vi "Fitting on a Sphere.vi"(3 "Z":dbl[](array[numeric]) format="%.2f", 4 "Y":dbl[](array[numeric]) format="%.2f", 5 "X":dbl[](array[numeric]) format="%.2f") -> (0 "error":i32, 1 "r":dbl format="%.2f", 2 "x0, y0, z0":dbl[](array[numeric]) format="%.2f")   [LabVIEW 2017, in "NI_Gmath.lvlib"]
doc: "Determines the best spherical fit on a cloud of points in 3D."
uses:
  <vilib>/gmath/NI_Gmath.lvlib
  <vilib>/Analysis/baseanly.llb/Mean (DBL).vi
  <vilib>/Analysis/7linalg.llb/Solve Linear Equations (single right hand).vi
  <vilib>/Analysis/baseanly.llb/Solve Linear Equations By Cholesky.vi
  <vilib>/Analysis/baseanly.llb/Real Matrix to Compact Array.vi
  <vilib>/Analysis/baseanly.llb/Real Compact Tri-Matrix Linear Eqs.vi
  <vilib>/Analysis/7linalg.llb/Solve Linear Eqs (General).vi
  <vilib>/Analysis/7linalg.llb/Solve Linear Eqs (Gen, single right hand).vi
  <vilib>/Analysis/NI_AALPro.lvlib
  <vilib>/Analysis/NI_AALBase.lvlib
panel:
  # "Example:\n\n X: data points\n Y: data points \n Z: data points"
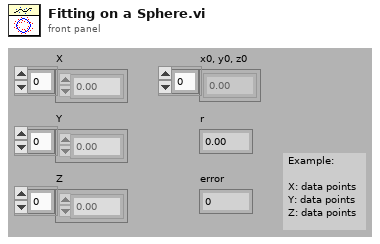
[diagram p1: front panel]
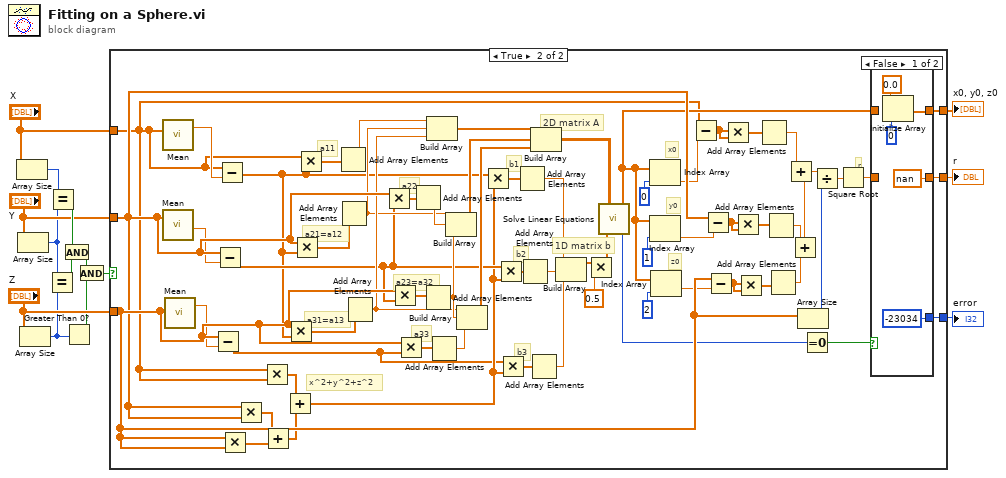
[diagram p0: block diagram]
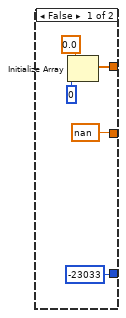
[diagram p2: hidden frame]
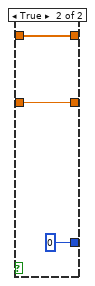
[diagram p3: hidden frame]
diagram:
  n1 = Array Size(array="X") -> (size(s)=w10:i32)
  n2 = Array Size(array="Y") -> (size(s)=w7:i32)
  n3 = Array Size(array="Z") -> (size(s)=w4:i32)
  n4 = Equal?(x=w7, y=w4) -> (x = y?=w5:bool)
  n5 = Equal?(x=w10, y=w7) -> (x = y?=w9:bool)
  n6 = And(x=w9, y=w5) -> (x .and. y?=w2:bool)
  n7 = Greater Than 0?(x=w4) -> (x > 0?=w3:bool)
  n8 = And(x=w2, y=w3) -> (x .and. y?=w1:bool)
  n9 = case shown="True" w1 {
    tunnel: "X" -> [_ w20]
    tunnel: "Z" -> [_ w81]
    tunnel: "Y" -> [_ w68]
    tunnel: [nan w26] -> w14
    tunnel: [w17 w24] -> w13
    tunnel: [-23033 w21] -> w12
    frame False {
      n10 = Initialize Array(0.0, 0) -> (w17:dbl[])
    }
    frame True {
      # "a11"
      # "a21=a12"
      # "a31=a13"
      # "a22"
      # "a23=a32"
      # "a33"
      # "x^2+y^2+z^2"
      # "b1"
      # "b2"
      # "b3"
      # "2D matrix A"
      # "1D matrix b"
      # "x0"
      # "y0"
      # "z0"
      # "r"
      n11 = call-poly <vilib>:"Mean.vi"("X"=w20) -> ("mean"=w28:dbl)  [unwired: 1 out]
      n12 = call-poly <vilib>:"Mean.vi"("X"=w68) -> ("mean"=w29:dbl)  [unwired: 1 out]
      n13 = call-poly <vilib>:"Mean.vi"("X"=w81) -> ("mean"=w30:dbl)  [unwired: 1 out]
      n14 = Subtract(x=w81, y=w30) -> (x-y=w36:dbl[])
      n15 = Subtract(x=w68, y=w29) -> (x-y=w42:dbl[])
      n16 = Subtract(x=w20, y=w28) -> (x-y=w35:dbl[])
      n17 = Multiply(x=w81, y=w81) -> (x*y=w32:dbl[])
      n18 = Multiply(x=w68, y=w68) -> (x*y=w31:dbl[])
      n19 = Multiply(x=w20, y=w20) -> (x*y=w34:dbl[])
      n20 = Add(x=w31, y=w32) -> (x+y=w33:dbl[])
      n21 = Add(x=w34, y=w33) -> (x+y=w37:dbl[])
      n22 = Multiply(x=w81, y=w35) -> (x*y=w41:dbl[])
      n23 = Multiply(x=w68, y=w35) -> (x*y=w40:dbl[])
      n24 = Multiply(x=w20, y=w35) -> (x*y=w38:dbl[])
      n25 = Add Array Elements(numeric array=w38) -> (sum=w39:dbl)
      n26 = Add Array Elements(numeric array=w40) -> (sum=w43:dbl)
      n27 = Add Array Elements(numeric array=w41) -> (sum=w47:dbl)
      n28 = Multiply(x=w68, y=w42) -> (x*y=w44:dbl[])
      n29 = Multiply(x=w81, y=w42) -> (x*y=w46:dbl[])
      n30 = Multiply(x=w81, y=w36) -> (x*y=w49:dbl[])
      n31 = Add Array Elements(numeric array=w44) -> (sum=w45:dbl)
      n32 = Add Array Elements(numeric array=w46) -> (sum=w48:dbl)
      n33 = Build Array(w39, w43, w47) -> (w51:dbl[])
      n34 = Add Array Elements(numeric array=w49) -> (sum=w50:dbl)
      n35 = Build Array(w43, w45, w48) -> (w52:dbl[])
      n36 = Build Array(w47, w48, w50) -> (w53:dbl[])
      n37 = Multiply(x=w35, y=w37) -> (x*y=w54:dbl[])
      n38 = Multiply(x=w42, y=w37) -> (x*y=w55:dbl[])
      n39 = Multiply(x=w36, y=w37) -> (x*y=w56:dbl[])
      n40 = Add Array Elements(numeric array=w54) -> (sum=w58:dbl)
      n41 = Add Array Elements(numeric array=w55) -> (sum=w59:dbl)
      n42 = Add Array Elements(numeric array=w56) -> (sum=w60:dbl)
      n43 = Build Array(w51, w52, w53) -> (w57:dbl[][])
      n44 = Build Array(w58, w59, w60) -> (w62:dbl[])
      n45 = Multiply(x=w62, y=0.5) -> (x*y=w84:dbl[])
      n46 = call-poly <vilib>:"Solve Linear Equations.vi"("Known Vector"=w84, "Input Matrix"=w57) -> ("error"=w23:i32, "Solution Vector"=w25:dbl[])  [unwired: 1 in]
      n47 = Index Array(array=w25, index=0) -> (element=w66:dbl)
      n48 = Index Array(array=w25, index=1) -> (element=w69:dbl)
      n49 = Index Array(array=w25, index=2) -> (element=w71:dbl)
      n50 = Subtract(x=w20, y=w66) -> (x-y=w67:dbl[])
      n51 = Subtract(x=w68, y=w69) -> (x-y=w70:dbl[])
      n52 = Subtract(x=w81, y=w71) -> (x-y=w72:dbl[])
      n53 = Multiply(x=w67, y=w67) -> (x*y=w73:dbl[])
      n54 = Multiply(x=w70, y=w70) -> (x*y=w74:dbl[])
      n55 = Multiply(x=w72, y=w72) -> (x*y=w75:dbl[])
      n56 = Add Array Elements(numeric array=w73) -> (sum=w79:dbl)
      n57 = Add Array Elements(numeric array=w74) -> (sum=w77:dbl)
      n58 = Add Array Elements(numeric array=w75) -> (sum=w76:dbl)
      n59 = Add(x=w77, y=w76) -> (x+y=w78:dbl)
      n60 = Add(x=w79, y=w78) -> (x+y=w80:dbl)
      n61 = Array Size(array=w81) -> (size(s)=w82:i32)
      n62 = Equal To 0?(x=w23) -> (x = 0?=w22:bool)
      n63 = Divide(x=w80, y=w82) -> (x/y=w83:dbl)
      n64 = Square Root(x=w83) -> (sqrt(x)=w27:dbl)
      n65 = case shown="False" w22 {
        tunnel: w27 -> [_ w92]
        tunnel: [nan w92] -> w26
        tunnel: w25 -> [_ w91]
        tunnel: [w87 w91] -> w24
        tunnel: [-23034 0] -> w21
        frame False {
          n66 = Initialize Array(0.0, 0) -> (w87:dbl[])
        }
        frame True {
        }
      }
    }
  }
  "r" <- w14
  "x0, y0, z0" <- w13
  "error" <- w12
